vi "Save Data.vi"(5 "Temperatura balero":dbl, 6 "Factor de potencia":dbl, 7 "Velocidad del motor":dbl, 8 "error in (no error)":errorcluster, 9 "Temperatura carcasa":dbl, 10 "Corriente":dbl, 11 "Voltaje":dbl) -> (0 "error out":errorcluster)   [LabVIEW 2020]
uses:
  <vilib>/drjdpowell/SQLite Library/SQL Connection/Open (path).vi
  <vilib>/drjdpowell/SQLite Library/SQL Connection/Open (string).vi
  <vilib>/AdvancedString/Path To Command Line String.vi
  <vilib>/drjdpowell/SQLite Library/SQL Connection/Execute SQL (No results).vi
  <vilib>/drjdpowell/SQLite Library/SQL Connection/Connection.lvclass
  <vilib>/drjdpowell/SQLite Library/SQLite.lvlib
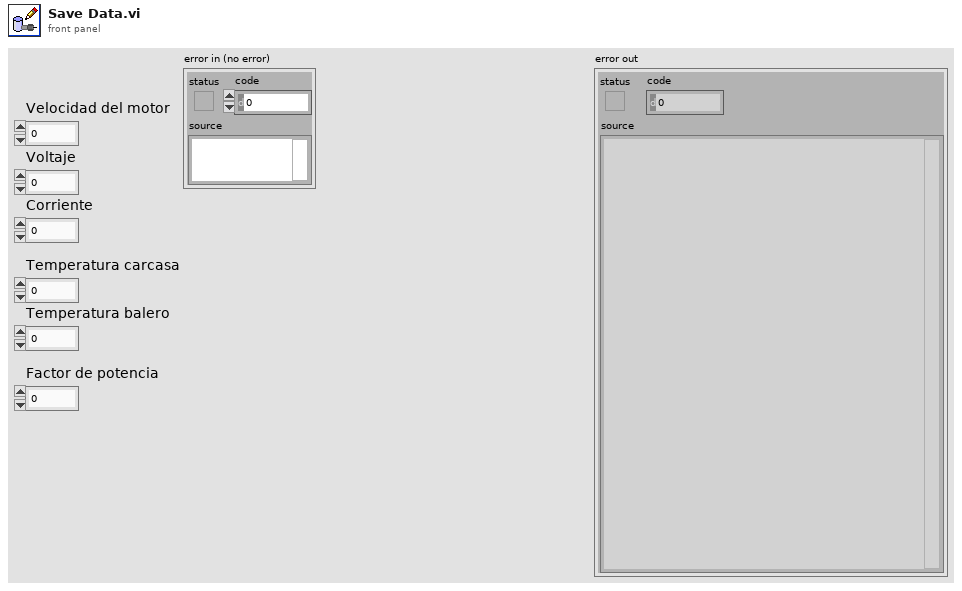
[diagram p1: front panel]
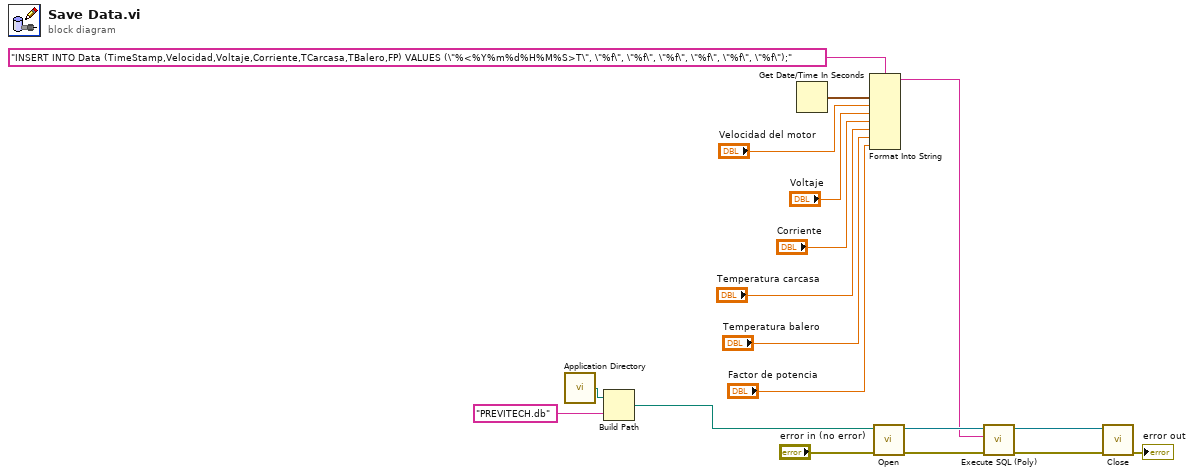
[diagram p0: block diagram]
diagram:
  n1 = call <vilib>:"Application Directory.vi"() -> ("Application Directory"=w4:path)
  n2 = Build Path(base path=w4, name or relative path="PREVITECH.db") -> (appended path=w2:path)
  n3 = Get Date/Time In Seconds() -> (seconds since 1Jan1904=w12:timestamp)
  n4 = Format Into String(format string="INSERT INTO Data (TimeStamp,Velocidad,Voltaje,Corriente,TCarcasa,TBalero,FP) VALUES (\"%<%Y%m%d%H%M%S>T\", \"%f\", \"%f\", \"%f\", \"%f\", \"%f\", \"%f\");", w12, "Velocidad del motor", "Voltaje", "Corriente", "Temperatura carcasa", "Temperatura balero", "Factor de potencia") -> (resulting string=w1:string)  [unwired: 2 in, 1 out]
  n5 = call-poly <vilib>:"Open.vi"("error in (no error)"="error in (no error)", "db file"=w2) -> ("error out"=w10:errorcluster, "SQLite Connection"=w6:refnum<class "Connection.lvclass">)  [unwired: 8 in]
  n6 = call-poly <vilib>:"Execute SQL (Poly).vi"("error in (no error)"=w10, "SQL"=w1, "SQLite Connection in"=w6) -> ("error out"=w9:errorcluster, "SQLite Connection"=w5:refnum<class "Connection.lvclass">)  [unwired: 7 in]
  n7 = call-dynamic "Close.vi"("error in (no error)"=w9, "SQLite Connection in"=w5) -> ("error out"=→"error out":errorcluster)  [unwired: 9 in]
